vi "Functional Global - Raw Inputs and Outputs.vi"(7 "Functional Global Operation (Read)":T1=enum."Read" caption="功能全局操作（读取）", 10 "Outputs in":dbl[](array[numeric]) caption="输出_输入", 11 "Inputs in":dbl[](array[numeric]) caption="输入_输入") -> (2 "Outputs out":dbl[](array[numeric]) caption="输出_输出", 3 "Inputs out":dbl[](array[numeric]) caption="输入_输出")   [LabVIEW 2013]
uses:
  controls/Functional Global Operation.ctl
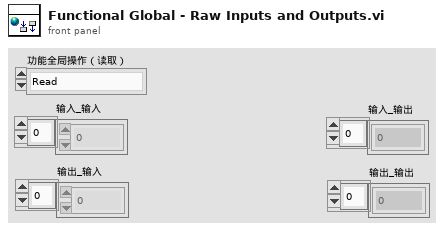
[diagram p1: front panel]
types:
  T1 = typedef "Functional Global Operation.ctl" = enum16{"Initialize", "Read", "Write"}
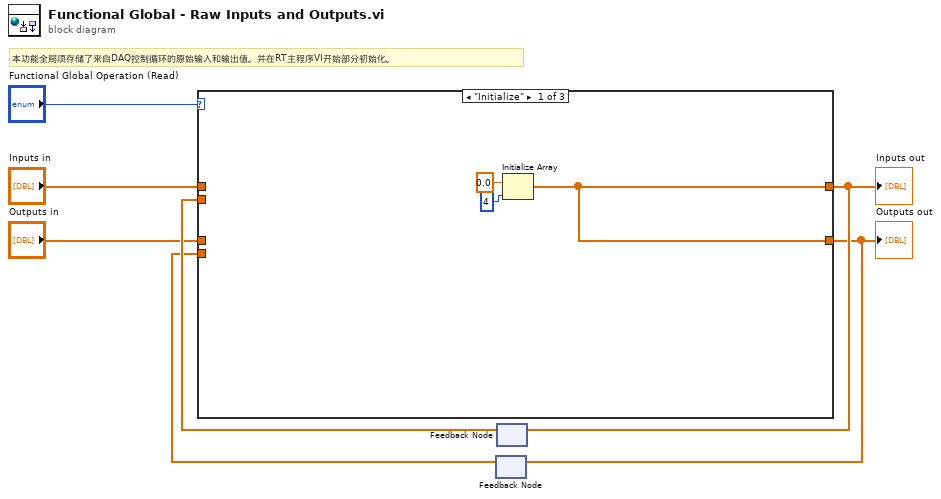
[diagram p0: block diagram]
diagram:
  # "本功能全局项存储了来自DAQ控制循环的原始输入和输出值。并在RT主程序VI开始部分初始化。"
  n1 = feedback #1() -> (w1:dbl[])  [unwired: 1 in]
  n2 = feedback #2() -> (w5:dbl[])  [unwired: 1 in]
  n3 = case shown="\"Initialize\"" "Functional Global Operation (Read)" {
    tunnel: "Inputs in" -> [_ _ w14]
    tunnel: [w8 w12 w14] -> w4
    tunnel: w5 -> [_ w12 _]
    tunnel: "Outputs in" -> [_ _ w13]
    tunnel: [w8 w11 w13] -> w2
    tunnel: w1 -> [_ w11 _]
    frame "Initialize" {
      n4 = Initialize Array(0.0 ("element"), 4 ("dimension size")) -> (w8:dbl[])
    }
    frame "Read", Default {
    }
    frame "Write" {
    }
  }
  "Inputs out" <- w4
  "Outputs out" <- w2
  n5 = feedback-in #1(w2) -> ()
  n6 = feedback-in #2(w4) -> ()
